vi "App - analyze RUS V6.vi"() -> ()   [LabVIEW 2018] (continued)
"file name str"="D:\\Data\\Ultrasound\\LSCO\\LSCO22__130814c\\5_Cooling_2nd_try\\September_2014\\091814\\14.56800K_500_2500_2.10000V_0.00000T_Sep18-2014__00-30-29_001_091814.bin", "mod time(min)"=58230990.483333334, "file format"=enum."binary", "power(V)"=2.1, "Magn Field(T) "=0.0}, {"temperature"=14.564, "temperature str"="14.56400", "file path"=path "D:/Data/Ultrasound/LSCO/LSCO22__130814c/5_Cooling_2nd_try/September_2014/091814/14.56400K_500_2500_2.10000V_0.00000T_Sep18-2014__00-31-48_001_091814.bin", "last mod"=timestamp(3493859508 s since 1904-01-01), "file name str"="D:\\Data\\Ultrasound\\LSCO\\LSCO22__130814c\\5_Cooling_2nd_try\\September_2014\\091814\\14.56400K_500_2500_2.10000V_0.00000T_Sep18-2014__00-31-48_001_091814.bin", "mod time(min)"=58230991.8, "file format"=enum."binary", "power(V)"=2.1, "Magn Field(T) "=0.0}, {"temperature"=14.565, "temperature str"="14.56500", "file path"=path "D:/Data/Ultrasound/LSCO/LSCO22__130814c/5_Cooling_2nd_try/September_2014/091814/14.56500K_500_2500_2.10000V_0.00000T_Sep18-2014__00-33-08_001_091814.bin", "last mod"=timestamp(3493859588 s since 1904-01-01), "file name str"="D:\\Data\\Ultrasound\\LSCO\\LSCO22__130814c\\5_Cooling_2nd_try\\September_2014\\091814\\14.56500K_500_2500_2.10000V_0.00000T_Sep18-2014__00-33-08_001_091814.bin", "mod time(min)"=58230993.13333333, "file format"=enum."binary", "power(V)"=2.1, "Magn Field(T) "=0.0}, {"temperature"=14.561, "temperature str"="14.56100", "file path"=path "D:/Data/Ultrasound/LSCO/LSCO22__130814c/5_Cooling_2nd_try/September_2014/091814/14.56100K_500_2500_2.10000V_0.00000T_Sep18-2014__00-34-27_001_091814.bin", "last mod"=timestamp(3493859667 s since 1904-01-01), "file name str"="D:\\Data\\Ultrasound\\LSCO\\LSCO22__130814c\\5_Cooling_2nd_try\\September_2014\\091814\\14.56100K_500_2500_2.10000V_0.00000T_Sep18-2014__00-34-27_001_091814.bin", "mod time(min)"=58230994.45, "file format"=enum."binary", "power(V)"=2.1, "Magn Field(T) "=0.0}, {"temperature"=14.557, "temperature str"="14.55700", "file path"=path "D:/Data/Ultrasound/LSCO/LSCO22__130814c/5_Cooling_2nd_try/September_2014/091814/14.55700K_500_2500_2.10000V_0.00000T_Sep18-2014__00-35-47_001_091814.bin", "last mod"=timestamp(3493859747 s since 1904-01-01), "file name str"="D:\\Data\\Ultrasound\\LSCO\\LSCO22__130814c\\5_Cooling_2nd_try\\September_2014\\091814\\14.55700K_500_2500_2.10000V_0.00000T_Sep18-2014__00-35-47_001_091814.bin", "mod time(min)"=58230995.78333333, "file format"=enum."binary", "power(V)"=2.1, "Magn Field(T) "=0.0}, {"temperature"=14.553, "temperature str"="14.55300", "file path"=path "D:/Data/Ultrasound/LSCO/LSCO22__130814c/5_Cooling_2nd_try/September_2014/091814/14.55300K_500_2500_2.10000V_0.00000T_Sep18-2014__00-37-06_001_091814.bin", "last mod"=timestamp(3493859826 s since 1904-01-01), "file name str"="D:\\Data\\Ultrasound\\LSCO\\LSCO22__130814c\\5_Cooling_2nd_try\\September_2014\\091814\\14.55300K_500_2500_2.10000V_0.00000T_Sep18-2014__00-37-06_001_091814.bin", "mod time(min)"=58230997.1, "file format"=enum."binary", "power(V)"=2.1, "Magn Field(T) "=0.0}, {"temperature"=14.55, "temperature str"="14.55000", "file path"=path "D:/Data/Ultrasound/LSCO/LSCO22__130814c/5_Cooling_2nd_try/September_2014/091814/14.55000K_500_2500_2.10000V_0.00000T_Sep18-2014__00-38-25_001_091814.bin", "last mod"=timestamp(3493859905 s since 1904-01-01), "file name str"="D:\\Data\\Ultrasound\\LSCO\\LSCO22__130814c\\5_Cooling_2nd_try\\September_2014\\091814\\14.55000K_500_2500_2.10000V_0.00000T_Sep18-2014__00-38-25_001_091814.bin", "mod time(min)"=58230998.416666664, "file format"=enum."binary", "power(V)"=2.1, "Magn Field(T) "=0.0}, {"temperature"=14.546, "temperature str"="14.54600", "file path"=path "D:/Data/Ultrasound/LSCO/LSCO22__130814c/5_Cooling_2nd_try/September_2014/091814/14.54600K_500_2500_2.10000V_0.00000T_Sep18-2014__00-39-45_001_091814.bin", "last mod"=timestamp(3493859985 s since 1904-01-01), "file name str"="D:\\Data\\Ultrasound\\LSCO\\LSCO22__130814c\\5_Cooling_2nd_try\\September_2014\\091814\\14.54600K_500_2500_2.10000V_0.00000T_Sep18-2014__00-39-45_001_091814.bin", "mod time(min)"=58230999.75, "file format"=enum."binary", "power(V)"=2.1, "Magn Field(T) "=0.0}, {"temperature"=14.543, "temperature str"="14.54300", "file path"=path "D:/Data/Ultrasound/LSCO/LSCO22__130814c/5_Cooling_2nd_try/September_2014/091814/14.54300K_500_2500_2.10000V_0.00000T_Sep18-2014__00-41-04_001_091814.bin", "last mod"=timestamp(3493860064 s since 1904-01-01), "file name str"="D:\\Data\\Ultrasound\\LSCO\\LSCO22__130814c\\5_Cooling_2nd_try\\September_2014\\091814\\14.54300K_500_2500_2.10000V_0.00000T_Sep18-2014__00-41-04_001_091814.bin", "mod time(min)"=58231001.06666667, "file format"=enum."binary", "power(V)"=2.1, "Magn Field(T) "=0.0}, {"temperature"=14.545, "temperature str"="14.54500", "file path"=path "D:/Data/Ultrasound/LSCO/LSCO22__130814c/5_Cooling_2nd_try/September_2014/091814/14.54500K_500_2500_2.10000V_0.00000T_Sep18-2014__00-42-24_001_091814.bin", "last mod"=timestamp(3493860144 s since 1904-01-01), "file name str"="D:\\Data\\Ultrasound\\LSCO\\LSCO22__130814c\\5_Cooling_2nd_try\\September_2014\\091814\\14.54500K_500_2500_2.10000V_0.00000T_Sep18-2014__00-42-24_001_091814.bin", "mod time(min)"=58231002.4, "file format"=enum."binary", "power(V)"=2.1, "Magn Field(T) "=0.0}, {"temperature"=14.546, "temperature str"="14.54600", "file path"=path "D:/Data/Ultrasound/LSCO/LSCO22__130814c/5_Cooling_2nd_try/September_2014/091814/14.54600K_500_2500_2.10000V_0.00000T_Sep18-2014__00-43-43_001_091814.bin", "last mod"=timestamp(3493860223 s since 1904-01-01), "file name str"="D:\\Data\\Ultrasound\\LSCO\\LSCO22__130814c\\5_Cooling_2nd_try\\September_2014\\091814\\14.54600K_500_2500_2.10000V_0.00000T_Sep18-2014__00-43-43_001_091814.bin", "mod time(min)"=58231003.71666667, "file format"=enum."binary", "power(V)"=2.1, "Magn Field(T) "=0.0}, {"temperature"=14.542, "temperature str"="14.54200", "file path"=path "D:/Data/Ultrasound/LSCO/LSCO22__130814c/5_Cooling_2nd_try/September_2014/091814/14.54200K_500_2500_2.10000V_0.00000T_Sep18-2014__00-45-02_001_091814.bin", "last mod"=timestamp(3493860302 s since 1904-01-01), "file name str"="D:\\Data\\Ultrasound\\LSCO\\LSCO22__130814c\\5_Cooling_2nd_try\\September_2014\\091814\\14.54200K_500_2500_2.10000V_0.00000T_Sep18-2014__00-45-02_001_091814.bin", "mod time(min)"=58231005.03333333, "file format"=enum."binary", "power(V)"=2.1, "Magn Field(T) "=0.0}, {"temperature"=14.545, "temperature str"="14.54500", "file path"=path "D:/Data/Ultrasound/LSCO/LSCO22__130814c/5_Cooling_2nd_try/September_2014/091814/14.54500K_500_2500_2.10000V_0.00000T_Sep18-2014__00-46-22_001_091814.bin", "last mod"=timestamp(3493860382 s since 1904-01-01), "file name str"="D:\\Data\\Ultrasound\\LSCO\\LSCO22__130814c\\5_Cooling_2nd_try\\September_2014\\091814\\14.54500K_500_2500_2.10000V_0.00000T_Sep18-2014__00-46-22_001_091814.bin", "mod time(min)"=58231006.36666667, "file format"=enum."binary", "power(V)"=2.1, "Magn Field(T) "=0.0}, {"temperature"=14.547, "temperature str"="14.54700", "file path"=path "D:/Data/Ultrasound/LSCO/LSCO22__130814c/5_Cooling_2nd_try/September_2014/091814/14.54700K_500_2500_2.10000V_0.00000T_Sep18-2014__00-47-41_001_091814.bin", "last mod"=timestamp(3493860461 s since 1904-01-01), "file name str"="D:\\Data\\Ultrasound\\LSCO\\LSCO22__130814c\\5_Cooling_2nd_try\\September_2014\\091814\\14.54700K_500_2500_2.10000V_0.00000T_Sep18-2014__00-47-41_001_091814.bin", "mod time(min)"=58231007.68333333, "file format"=enum."binary", "power(V)"=2.1, "Magn Field(T) "=0.0}, {"temperature"=14.544, "temperature str"="14.54400", "file path"=path "D:/Data/Ultrasound/LSCO/LSCO22__130814c/5_Cooling_2nd_try/September_2014/091814/14.54400K_500_2500_2.10000V_0.00000T_Sep18-2014__00-49-00_001_091814.bin", "last mod"=timestamp(3493860540 s since 1904-01-01), "file name str"="D:\\Data\\Ultrasound\\LSCO\\LSCO22__130814c\\5_Cooling_2nd_try\\September_2014\\091814\\14.54400K_500_2500_2.10000V_0.00000T_Sep18-2014__00-49-00_001_091814.bin", "mod time(min)"=58231009.0, "file format"=enum."binary", "power(V)"=2.1, "Magn Field(T) "=0.0}, {"temperature"=14.538, "temperature str"="14.53800", "file path"=path "D:/Data/Ultrasound/LSCO/LSCO22__130814c/5_Cooling_2nd_try/September_2014/091814/14.53800K_500_2500_2.10000V_0.00000T_Sep18-2014__00-50-20_001_091814.bin", "last mod"=timestamp(3493860620 s since 1904-01-01), "file name str"="D:\\Data\\Ultrasound\\LSCO\\LSCO22__130814c\\5_Cooling_2nd_try\\September_2014\\091814\\14.53800K_500_2500_2.10000V_0.00000T_Sep18-2014__00-50-20_001_091814.bin", "mod time(min)"=58231010.333333336, "file format"=enum."binary", "power(V)"=2.1, "Magn Field(T) "=0.0}, {"temperature"=14.537, "temperature str"="14.53700", "file path"=path "D:/Data/Ultrasound/LSCO/LSCO22__130814c/5_Cooling_2nd_try/September_2014/091814/14.53700K_500_2500_2.10000V_0.00000T_Sep18-2014__00-51-39_001_091814.bin", "last mod"=timestamp(3493860699 s since 1904-01-01), "file name str"="D:\\Data\\Ultrasound\\LSCO\\LSCO22__130814c\\5_Cooling_2nd_try\\September_2014\\091814\\14.53700K_500_2500_2.10000V_0.00000T_Sep18-2014__00-51-39_001_091814.bin", "mod time(min)"=58231011.65, "file format"=enum."binary", "power(V)"=2.1, "Magn Field(T) "=0.0}, {"temperature"=14.527, "temperature str"="14.52700", "file path"=path "D:/Data/Ultrasound/LSCO/LSCO22__130814c/5_Cooling_2nd_try/September_2014/091814/14.52700K_500_2500_2.10000V_0.00000T_Sep18-2014__00-52-59_001_091814.bin", "last mod"=timestamp(3493860779 s since 1904-01-01), "file name str"="D:\\Data\\Ultrasound\\LSCO\\LSCO22__130814c\\5_Cooling_2nd_try\\September_2014\\091814\\14.52700K_500_2500_2.10000V_0.00000T_Sep18-2014__00-52-59_001_091814.bin", "mod time(min)"=58231012.983333334, "file format"=enum."binary", "power(V)"=2.1, "Magn Field(T) "=0.0}, {"temperature"=14.532, "temperature str"="14.53200", "file path"=path "D:/Data/Ultrasound/LSCO/LSCO22__130814c/5_Cooling_2nd_try/September_2014/091814/14.53200K_500_2500_2.10000V_0.00000T_Sep18-2014__00-54-18_001_091814.bin", "last mod"=timestamp(3493860858 s since 1904-01-01), "file name str"="D:\\Data\\Ultrasound\\LSCO\\LSCO22__130814c\\5_Cooling_2nd_try\\September_2014\\091814\\14.53200K_500_2500_2.10000V_0.00000T_Sep18-2014__00-54-18_001_091814.bin", "mod time(min)"=58231014.3, "file format"=enum."binary", "power(V)"=2.1, "Magn Field(T) "=0.0}, {"temperature"=14.532, "temperature str"="14.53200", "file path"=path "D:/Data/Ultrasound/LSCO/LSCO22__130814c/5_Cooling_2nd_try/September_2014/091814/14.53200K_500_2500_2.10000V_0.00000T_Sep18-2014__00-55-37_001_091814.bin", "last mod"=timestamp(3493860937 s since 1904-01-01), "file name str"="D:\\Data\\Ultrasound\\LSCO\\LSCO22__130814c\\5_Cooling_2nd_try\\September_2014\\091814\\14.53200K_500_2500_2.10000V_0.00000T_Sep18-2014__00-55-37_001_091814.bin", "mod time(min)"=58231015.61666667, "file format"=enum."binary", "power(V)"=2.1, "Magn Field(T) "=0.0}, {"temperature"=14.525, "temperature str"="14.52500", "file path"=path "D:/Data/Ultrasound/LSCO/LSCO22__130814c/5_Cooling_2nd_try/September_2014/091814/14.52500K_500_2500_2.10000V_0.00000T_Sep18-2014__00-56-57_001_091814.bin", "last mod"=timestamp(3493861017 s since 1904-01-01), "file name str"="D:\\Data\\Ultrasound\\LSCO\\LSCO22__130814c\\5_Cooling_2nd_try\\September_2014\\091814\\14.52500K_500_2500_2.10000V_0.00000T_Sep18-2014__00-56-57_001_091814.bin", "mod time(min)"=58231016.95, "file format"=enum."binary", "power(V)"=2.1, "Magn Field(T) "=0.0}, {"temperature"=14.52, "temperature str"="14.52000", "file path"=path "D:/Data/Ultrasound/LSCO/LSCO22__130814c/5_Cooling_2nd_try/September_2014/091814/14.52000K_500_2500_2.10000V_0.00000T_Sep18-2014__00-58-16_001_091814.bin", "last mod"=timestamp(3493861096 s since 1904-01-01), "file name str"="D:\\Data\\Ultrasound\\LSCO\\LSCO22__130814c\\5_Cooling_2nd_try\\September_2014\\091814\\14.52000K_500_2500_2.10000V_0.00000T_Sep18-2014__00-58-16_001_091814.bin", "mod time(min)"=58231018.266666666, "file format"=enum."binary", "power(V)"=2.1, "Magn Field(T) "=0.0}, {"temperature"=14.519, "temperature str"="14.51900", "file path"=path "D:/Data/Ultrasound/LSCO/LSCO22__130814c/5_Cooling_2nd_try/September_2014/091814/14.51900K_500_2500_2.10000V_0.00000T_Sep18-2014__00-59-35_001_091814.bin", "last mod"=timestamp(3493861175 s since 1904-01-01), "file name str"="D:\\Data\\Ultrasound\\LSCO\\LSCO22__130814c\\5_Cooling_2nd_try\\September_2014\\091814\\14.51900K_500_2500_2.10000V_0.00000T_Sep18-2014__00-59-35_001_091814.bin", "mod time(min)"=58231019.583333336, "file format"=enum."binary", "power(V)"=2.1, "Magn Field(T) "=0.0}, {"temperature"=14.515, "temperature str"="14.51500", "file path"=path "D:/Data/Ultrasound/LSCO/LSCO22__130814c/5_Cooling_2nd_try/September_2014/091814/14.51500K_500_2500_2.10000V_0.00000T_Sep18-2014__01-00-55_001_091814.bin", "last mod"=timestamp(3493861255 s since 1904-01-01), "file name str"="D:\\Data\\Ultrasound\\LSCO\\LSCO22__130814c\\5_Cooling_2nd_try\\September_2014\\091814\\14.51500K_500_2500_2.10000V_0.00000T_Sep18-2014__01-00-55_001_091814.bin", "mod time(min)"=58231020.916666664, "file format"=enum."binary", "power(V)"=2.1, "Magn Field(T) "=0.0}, {"temperature"=14.515, "temperature str"="14.51500", "file path"=path "D:/Data/Ultrasound/LSCO/LSCO22__130814c/5_Cooling_2nd_try/September_2014/091814/14.51500K_500_2500_2.10000V_0.00000T_Sep18-2014__01-02-14_001_091814.bin", "last mod"=timestamp(3493861334 s since 1904-01-01), "file name str"="D:\\Data\\Ultrasound\\LSCO\\LSCO22__130814c\\5_Cooling_2nd_try\\September_2014\\091814\\14.51500K_500_2500_2.10000V_0.00000T_Sep18-2014__01-02-14_001_091814.bin", "mod time(min)"=58231022.233333334, "file format"=enum."binary", "power(V)"=2.1, "Magn Field(T) "=0.0}, {"temperature"=14.511, "temperature str"="14.51100", "file path"=path "D:/Data/Ultrasound/LSCO/LSCO22__130814c/5_Cooling_2nd_try/September_2014/091814/14.51100K_500_2500_2.10000V_0.00000T_Sep18-2014__01-03-34_001_091814.bin", "last mod"=timestamp(3493861414 s since 1904-01-01), "file name str"="D:\\Data\\Ultrasound\\LSCO\\LSCO22__130814c\\5_Cooling_2nd_try\\September_2014\\091814\\14.51100K_500_2500_2.10000V_0.00000T_Sep18-2014__01-03-34_001_091814.bin", "mod time(min)"=58231023.56666667, "file format"=enum."binary", "power(V)"=2.1, "Magn Field(T) "=0.0}, {"temperature"=14.506, "temperature str"="14.50600", "file path"=path "D:/Data/Ultrasound/LSCO/LSCO22__130814c/5_Cooling_2nd_try/September_2014/091814/14.50600K_500_2500_2.10000V_0.00000T_Sep18-2014__01-04-53_001_091814.bin", "last mod"=timestamp(3493861493 s since 1904-01-01), "file name str"="D:\\Data\\Ultrasound\\LSCO\\LSCO22__130814c\\5_Cooling_2nd_try\\September_2014\\091814\\14.50600K_500_2500_2.10000V_0.00000T_Sep18-2014__01-04-53_001_091814.bin", "mod time(min)"=58231024.88333333, "file format"=enum."binary", "power(V)"=2.1, "Magn Field(T) "=0.0}, {"temperature"=14.507, "temperature str"="14.50700", "file path"=path "D:/Data/Ultrasound/LSCO/LSCO22__130814c/5_Cooling_2nd_try/September_2014/091814/14.50700K_500_2500_2.10000V_0.00000T_Sep18-2014__01-06-12_001_091814.bin", "last mod"=timestamp(3493861572 s since 1904-01-01), "file name str"="D:\\Data\\Ultrasound\\LSCO\\LSCO22__130814c\\5_Cooling_2nd_try\\September_2014\\091814\\14.50700K_500_2500_2.10000V_0.00000T_Sep18-2014__01-06-12_001_091814.bin", "mod time(min)"=58231026.2, "file format"=enum."binary", "power(V)"=2.1, "Magn Field(T) "=0.0}, {"temperature"=14.503, "temperature str"="14.50300", "file path"=path "D:/Data/Ultrasound/LSCO/LSCO22__130814c/5_Cooling_2nd_try/September_2014/091814/14.50300K_500_2500_2.10000V_0.00000T_Sep18-2014__01-07-32_001_091814.bin", "last mod"=timestamp(3493861652 s since 1904-01-01), "file name str"="D:\\Data\\Ultrasound\\LSCO\\LSCO22__130814c\\5_Cooling_2nd_try\\September_2014\\091814\\14.50300K_500_2500_2.10000V_0.00000T_Sep18-2014__01-07-32_001_091814.bin", "mod time(min)"=58231027.53333333, "file format"=enum."binary", "power(V)"=2.1, "Magn Field(T) "=0.0}, {"temperature"=14.501, "temperature str"="14.50100", "file path"=path "D:/Data/Ultrasound/LSCO/LSCO22__130814c/5_Cooling_2nd_try/September_2014/091814/14.50100K_500_2500_2.10000V_0.00000T_Sep18-2014__01-08-51_001_091814.bin", "last mod"=timestamp(3493861731 s since 1904-01-01), "file name str"="D:\\Data\\Ultrasound\\LSCO\\LSCO22__130814c\\5_Cooling_2nd_try\\September_2014\\091814\\14.50100K_500_2500_2.10000V_0.00000T_Sep18-2014__01-08-51_001_091814.bin", "mod time(min)"=58231028.85, "file format"=enum."binary", "power(V)"=2.1, "Magn Field(T) "=0.0}, {"temperature"=14.5, "temperature str"="14.50000", "file path"=path "D:/Data/Ultrasound/LSCO/LSCO22__130814c/5_Cooling_2nd_try/September_2014/091814/14.50000K_500_2500_2.10000V_0.00000T_Sep18-2014__01-10-11_001_091814.bin", "last mod"=timestamp(3493861811 s since 1904-01-01), "file name str"="D:\\Data\\Ultrasound\\LSCO\\LSCO22__130814c\\5_Cooling_2nd_try\\September_2014\\091814\\14.50000K_500_2500_2.10000V_0.00000T_Sep18-2014__01-10-11_001_091814.bin", "mod time(min)"=58231030.18333333, "file format"=enum."binary", "power(V)"=2.1, "Magn Field(T) "=0.0}, {"temperature"=14.504, "temperature str"="14.50400", "file path"=path "D:/Data/Ultrasound/LSCO/LSCO22__130814c/5_Cooling_2nd_try/September_2014/091814/14.50400K_500_2500_2.10000V_0.00000T_Sep18-2014__01-11-30_001_091814.bin", "last mod"=timestamp(3493861890 s since 1904-01-01), "file name str"="D:\\Data\\Ultrasound\\LSCO\\LSCO22__130814c\\5_Cooling_2nd_try\\September_2014\\091814\\14.50400K_500_2500_2.10000V_0.00000T_Sep18-2014__01-11-30_001_091814.bin", "mod time(min)"=58231031.5, "file format"=enum."binary", "power(V)"=2.1, "Magn Field(T) "=0.0}, {"temperature"=14.504, "temperature str"="14.50400", "file path"=path "D:/Data/Ultrasound/LSCO/LSCO22__130814c/5_Cooling_2nd_try/September_2014/091814/14.50400K_500_2500_2.10000V_0.00000T_Sep18-2014__01-12-49_001_091814.bin", "last mod"=timestamp(3493861969 s since 1904-01-01), "file name str"="D:\\Data\\Ultrasound\\LSCO\\LSCO22__130814c\\5_Cooling_2nd_try\\September_2014\\091814\\14.50400K_500_2500_2.10000V_0.00000T_Sep18-2014__01-12-49_001_091814.bin", "mod time(min)"=58231032.81666667, "file format"=enum."binary", "power(V)"=2.1, "Magn Field(T) "=0.0}, {"temperature"=14.507, "temperature str"="14.50700", "file path"=path "D:/Data/Ultrasound/LSCO/LSCO22__130814c/5_Cooling_2nd_try/September_2014/091814/14.50700K_500_2500_2.10000V_0.00000T_Sep18-2014__01-14-09_001_091814.bin", "last mod"=timestamp(3493862049 s since 1904-01-01), "file name str"="D:\\Data\\Ultrasound\\LSCO\\LSCO22__130814c\\5_Cooling_2nd_try\\September_2014\\091814\\14.50700K_500_2500_2.10000V_0.00000T_Sep18-2014__01-14-09_001_091814.bin", "mod time(min)"=58231034.15, "file format"=enum."binary", "power(V)"=2.1, "Magn Field(T) "=0.0}, {"temperature"=14.502, "temperature str"="14.50200", "file path"=path "D:/Data/Ultrasound/LSCO/LSCO22__130814c/5_Cooling_2nd_try/September_2014/091814/14.50200K_500_2500_2.10000V_0.00000T_Sep18-2014__01-15-28_001_091814.bin", "last mod"=timestamp(3493862128 s since 1904-01-01), "file name str"="D:\\Data\\Ultrasound\\LSCO\\LSCO22__130814c\\5_Cooling_2nd_try\\September_2014\\091814\\14.50200K_500_2500_2.10000V_0.00000T_Sep18-2014__01-15-28_001_091814.bin", "mod time(min)"=58231035.46666667, "file format"=enum."binary", "power(V)"=2.1, "Magn Field(T) "=0.0}, {"temperature"=14.501, "temperature str"="14.50100", "file path"=path "D:/Data/Ultrasound/LSCO/LSCO22__130814c/5_Cooling_2nd_try/September_2014/091814/14.50100K_500_2500_2.10000V_0.00000T_Sep18-2014__01-16-47_001_091814.bin", "last mod"=timestamp(3493862207 s since 1904-01-01), "file name str"="D:\\Data\\Ultrasound\\LSCO\\LSCO22__130814c\\5_Cooling_2nd_try\\September_2014\\091814\\14.50100K_500_2500_2.10000V_0.00000T_Sep18-2014__01-16-47_001_091814.bin", "mod time(min)"=58231036.78333333, "file format"=enum."binary", "power(V)"=2.1, "Magn Field(T) "=0.0}, {"temperature"=14.503, "temperature str"="14.50300", "file path"=path "D:/Data/Ultrasound/LSCO/LSCO22__130814c/5_Cooling_2nd_try/September_2014/091814/14.50300K_500_2500_2.10000V_0.00000T_Sep18-2014__01-18-07_001_091814.bin", "last mod"=timestamp(3493862287 s since 1904-01-01), "file name str"="D:\\Data\\Ultrasound\\LSCO\\LSCO22__130814c\\5_Cooling_2nd_try\\September_2014\\091814\\14.50300K_500_2500_2.10000V_0.00000T_Sep18-2014__01-18-07_001_091814.bin", "mod time(min)"=58231038.11666667, "file format"=enum."binary", "power(V)"=2.1, "Magn Field(T) "=0.0}, {"temperature"=14.496, "temperature str"="14.49600", "file path"=path "D:/Data/Ultrasound/LSCO/LSCO22__130814c/5_Cooling_2nd_try/September_2014/091814/14.49600K_500_2500_2.10000V_0.00000T_Sep18-2014__01-19-26_001_091814.bin", "last mod"=timestamp(3493862366 s since 1904-01-01), "file name str"="D:\\Data\\Ultrasound\\LSCO\\LSCO22__130814c\\5_Cooling_2nd_try\\September_2014\\091814\\14.49600K_500_2500_2.10000V_0.00000T_Sep18-2014__01-19-26_001_091814.bin", "mod time(min)"=58231039.43333333, "file format"=enum."binary", "power(V)"=2.1, "Magn Field(T) "=0.0}, {"temperature"=14.494, "temperature str"="14.49400", "file path"=path "D:/Data/Ultrasound/LSCO/LSCO22__130814c/5_Cooling_2nd_try/September_2014/091814/14.49400K_500_2500_2.10000V_0.00000T_Sep18-2014__01-20-46_001_091814.bin", "last mod"=timestamp(3493862446 s since 1904-01-01), "file name str"="D:\\Data\\Ultrasound\\LSCO\\LSCO22__130814c\\5_Cooling_2nd_try\\September_2014\\091814\\14.49400K_500_2500_2.10000V_0.00000T_Sep18-2014__01-20-46_001_091814.bin", "mod time(min)"=58231040.766666666, "file format"=enum."binary", "power(V)"=2.1, "Magn Field(T) "=0.0}, {"temperature"=14.494, "temperature str"="14.49400", "file path"=path "D:/Data/Ultrasound/LSCO/LSCO22__130814c/5_Cooling_2nd_try/September_2014/091814/14.49400K_500_2500_2.10000V_0.00000T_Sep18-2014__01-22-05_001_091814.bin", "last mod"=timestamp(3493862525 s since 1904-01-01), "file name str"="D:\\Data\\Ultrasound\\LSCO\\LSCO22__130814c\\5_Cooling_2nd_try\\September_2014\\091814\\14.49400K_500_2500_2.10000V_0.00000T_Sep18-2014__01-22-05_001_091814.bin", "mod time(min)"=58231042.083333336, "file format"=enum."binary", "power(V)"=2.1, "Magn Field(T) "=0.0}, {"temperature"=14.485, "temperature str"="14.48500", "file path"=path "D:/Data/Ultrasound/LSCO/LSCO22__130814c/5_Cooling_2nd_try/September_2014/091814/14.48500K_500_2500_2.10000V_0.00000T_Sep18-2014__01-23-24_001_091814.bin", "last mod"=timestamp(3493862604 s since 1904-01-01), "file name str"="D:\\Data\\Ultrasound\\LSCO\\LSCO22__130814c\\5_Cooling_2nd_try\\September_2014\\091814\\14.48500K_500_2500_2.10000V_0.00000T_Sep18-2014__01-23-24_001_091814.bin", "mod time(min)"=58231043.4, "file format"=enum."binary", "power(V)"=2.1, "Magn Field(T) "=0.0}, {"temperature"=14.485, "temperature str"="14.48500", "file path"=path "D:/Data/Ultrasound/LSCO/LSCO22__130814c/5_Cooling_2nd_try/September_2014/091814/14.48500K_500_2500_2.10000V_0.00000T_Sep18-2014__01-24-44_001_091814.bin", "last mod"=timestamp(3493862684 s since 1904-01-01), "file name str"="D:\\Data\\Ultrasound\\LSCO\\LSCO22__130814c\\5_Cooling_2nd_try\\September_2014\\091814\\14.48500K_500_2500_2.10000V_0.00000T_Sep18-2014__01-24-44_001_091814.bin", "mod time(min)"=58231044.733333334, "file format"=enum."binary", "power(V)"=2.1, "Magn Field(T) "=0.0}, {"temperature"=14.487, "temperature str"="14.48700", "file path"=path "D:/Data/Ultrasound/LSCO/LSCO22__130814c/5_Cooling_2nd_try/September_2014/091814/14.48700K_500_2500_2.10000V_0.00000T_Sep18-2014__01-26-03_001_091814.bin", "last mod"=timestamp(3493862763 s since 1904-01-01), "file name str"="D:\\Data\\Ultrasound\\LSCO\\LSCO22__130814c\\5_Cooling_2nd_try\\September_2014\\091814\\14.48700K_500_2500_2.10000V_0.00000T_Sep18-2014__01-26-03_001_091814.bin", "mod time(min)"=58231046.05, "file format"=enum."binary", "power(V)"=2.1, "Magn Field(T) "=0.0}, {"temperature"=14.486, "temperature str"="14.48600", "file path"=path "D:/Data/Ultrasound/LSCO/LSCO22__130814c/5_Cooling_2nd_try/September_2014/091814/14.48600K_500_2500_2.10000V_0.00000T_Sep18-2014__01-27-22_001_091814.bin", "last mod"=timestamp(3493862842 s since 1904-01-01), "file name str"="D:\\Data\\Ultrasound\\LSCO\\LSCO22__130814c\\5_Cooling_2nd_try\\September_2014\\091814\\14.48600K_500_2500_2.10000V_0.00000T_Sep18-2014__01-27-22_001_091814.bin", "mod time(min)"=58231047.36666667, "file format"=enum."binary", "power(V)"=2.1, "Magn Field(T) "=0.0}, {"temperature"=14.479, "temperature str"="14.47900", "file path"=path "D:/Data/Ultrasound/LSCO/LSCO22__130814c/5_Cooling_2nd_try/September_2014/091814/14.47900K_500_2500_2.10000V_0.00000T_Sep18-2014__01-28-42_001_091814.bin", "last mod"=timestamp(3493862922 s since 1904-01-01), "file name str"="D:\\Data\\Ultrasound\\LSCO\\LSCO22__130814c\\5_Cooling_2nd_try\\September_2014\\091814\\14.47900K_500_2500_2.10000V_0.00000T_Sep18-2014__01-28-42_001_091814.bin", "mod time(min)"=58231048.7, "file format"=enum."binary", "power(V)"=2.1, "Magn Field(T) "=0.0}, {"temperature"=14.477, "temperature str"="14.47700", "file path"=path "D:/Data/Ultrasound/LSCO/LSCO22__130814c/5_Cooling_2nd_try/September_2014/091814/14.47700K_500_2500_2.10000V_0.00000T_Sep18-2014__01-30-01_001_091814.bin", "last mod"=timestamp(3493863001 s since 1904-01-01), "file name str"="D:\\Data\\Ultrasound\\LSCO\\LSCO22__130814c\\5_Cooling_2nd_try\\September_2014\\091814\\14.47700K_500_2500_2.10000V_0.00000T_Sep18-2014__01-30-01_001_091814.bin", "mod time(min)"=58231050.016666666, "file format"=enum."binary", "power(V)"=2.1, "Magn Field(T) "=0.0}, {"temperature"=14.476, "temperature str"="14.47600", "file path"=path "D:/Data/Ultrasound/LSCO/LSCO22__130814c/5_Cooling_2nd_try/September_2014/091814/14.47600K_500_2500_2.10000V_0.00000T_Sep18-2014__01-31-21_001_091814.bin", "last mod"=timestamp(3493863081 s since 1904-01-01), "file name str"="D:\\Data\\Ultrasound\\LSCO\\LSCO22__130814c\\5_Cooling_2nd_try\\September_2014\\091814\\14.47600K_500_2500_2.10000V_0.00000T_Sep18-2014__01-31-21_001_091814.bin", "mod time(min)"=58231051.35, "file format"=enum."binary", "power(V)"=2.1, "Magn Field(T) "=0.0}, {"temperature"=14.474, "temperature str"="14.47400", "file path"=path "D:/Data/Ultrasound/LSCO/LSCO22__130814c/5_Cooling_2nd_try/September_2014/091814/14.47400K_500_2500_2.10000V_0.00000T_Sep18-2014__01-32-40_001_091814.bin", "last mod"=timestamp(3493863160 s since 1904-01-01), "file name str"="D:\\Data\\Ultrasound\\LSCO\\LSCO22__130814c\\5_Cooling_2nd_try\\September_2014\\091814\\14.47400K_500_2500_2.10000V_0.00000T_Sep18-2014__01-32-40_001_091814.bin", "mod time(min)"=58231052.666666664, "file format"=enum."binary", "power(V)"=2.1, "Magn Field(T) "=0.0}, {"temperature"=14.473, "temperature str"="14.47300", "file path"=path "D:/Data/Ultrasound/LSCO/LSCO22__130814c/5_Cooling_2nd_try/September_2014/091814/14.47300K_500_2500_2.10000V_0.00000T_Sep18-2014__01-33-59_001_091814.bin", "last mod"=timestamp(3493863239 s since 1904-01-01), "file name str"="D:\\Data\\Ultrasound\\LSCO\\LSCO22__130814c\\5_Cooling_2nd_try\\September_2014\\091814\\14.47300K_500_2500_2.10000V_0.00000T_Sep18-2014__01-33-59_001_091814.bin", "mod time(min)"=58231053.983333334, "file format"=enum."binary", "power(V)"=2.1, "Magn Field(T) "=0.0}, {"temperature"=14.478, "temperature str"="14.47800", "file path"=path "D:/Data/Ultrasound/LSCO/LSCO22__130814c/5_Cooling_2nd_try/September_2014/091814/14.47800K_500_2500_2.10000V_0.00000T_Sep18-2014__01-35-19_001_091814.bin", "last mod"=timestamp(3493863319 s since 1904-01-01), "file name str"="D:\\Data\\Ultrasound\\LSCO\\LSCO22__130814c\\5_Cooling_2nd_try\\September_2014\\091814\\14.47800K_500_2500_2.10000V_0.00000T_Sep18-2014__01-35-19_001_091814.bin", "mod time(min)"=58231055.31666667, "file format"=enum."binary", "power(V)"=2.1, "Magn Field(T) "=0.0}, {"temperature"=14.475, "temperature str"="14.47500", "file path"=path "D:/Data/Ultrasound/LSCO/LSCO22__130814c/5_Cooling_2nd_try/September_2014/091814/14.47500K_500_2500_2.10000V_0.00000T_Sep18-2014__01-36-38_001_091814.bin", "last mod"=timestamp(3493863398 s since 1904-01-01), "file name str"="D:\\Data\\Ultrasound\\LSCO\\LSCO22__130814c\\5_Cooling_2nd_try\\September_2014\\091814\\14.47500K_500_2500_2.10000V_0.00000T_Sep18-2014__01-36-38_001_091814.bin", "mod time(min)"=58231056.63333333, "file format"=enum."binary", "power(V)"=2.1, "Magn Field(T) "=0.0}, {"temperature"=14.47, "temperature str"="14.47000", "file path"=path "D:/Data/Ultrasound/LSCO/LSCO22__130814c/5_Cooling_2nd_try/September_2014/091814/14.47000K_500_2500_2.10000V_0.00000T_Sep18-2014__01-37-58_001_091814.bin", "last mod"=timestamp(3493863478 s since 1904-01-01), "file name str"="D:\\Data\\Ultrasound\\LSCO\\LSCO22__130814c\\5_Cooling_2nd_try\\September_2014\\091814\\14.47000K_500_2500_2.10000V_0.00000T_Sep18-2014__01-37-58_001_091814.bin", "mod time(min)"=58231057.96666667, "file format"=enum."binary", "power(V)"=2.1, "Magn Field(T) "=0.0}, {"temperature"=14.472, "temperature str"="14.47200", "file path"=path "D:/Data/Ultrasound/LSCO/LSCO22__130814c/5_Cooling_2nd_try/September_2014/091814/14.47200K_500_2500_2.10000V_0.00000T_Sep18-2014__01-39-17_001_091814.bin", "last mod"=timestamp(3493863557 s since 1904-01-01), "file name str"="D:\\Data\\Ultrasound\\LSCO\\LSCO22__130814c\\5_Cooling_2nd_try\\September_2014\\091814\\14.47200K_500_2500_2.10000V_0.00000T_Sep18-2014__01-39-17_001_091814.bin", "mod time(min)"=58231059.28333333, "file format"=enum."binary", "power(V)"=2.1, "Magn Field(T) "=0.0}, {"temperature"=14.471, "temperature str"="14.47100", "file path"=path "D:/Data/Ultrasound/LSCO/LSCO22__130814c/5_Cooling_2nd_try/September_2014/091814/14.47100K_500_2500_2.10000V_0.00000T_Sep18-2014__01-40-36_001_091814.bin", "last mod"=timestamp(3493863636 s since 1904-01-01), "file name str"="D:\\Data\\Ultrasound\\LSCO\\LSCO22__130814c\\5_Cooling_2nd_try\\September_2014\\091814\\14.47100K_500_2500_2.10000V_0.00000T_Sep18-2014__01-40-36_001_091814.bin", "mod time(min)"=58231060.6, "file format"=enum."binary", "power(V)"=2.1, "Magn Field(T) "=0.0}, {"temperature"=14.469, "temperature str"="14.46900", "file path"=path "D:/Data/Ultrasound/LSCO/LSCO22__130814c/5_Cooling_2nd_try/September_2014/091814/14.46900K_500_2500_2.10000V_0.00000T_Sep18-2014__01-41-56_001_091814.bin", "last mod"=timestamp(3493863716 s since 1904-01-01), "file name str"="D:\\Data\\Ultrasound\\LSCO\\LSCO22__130814c\\5_Cooling_2nd_try\\September_2014\\091814\\14.46900K_500_2500_2.10000V_0.00000T_Sep18-2014__01-41-56_001_091814.bin", "mod time(min)"=58231061.93333333, "file format"=enum."binary", "power(V)"=2.1, "Magn Field(T) "=0.0}, {"temperature"=14.466, "temperature str"="14.46600", "file path"=path "D:/Data/Ultrasound/LSCO/LSCO22__130814c/5_Cooling_2nd_try/September_2014/091814/14.46600K_500_2500_2.10000V_0.00000T_Sep18-2014__01-43-15_001_091814.bin", "last mod"=timestamp(3493863795 s since 1904-01-01), "file name str"="D:\\Data\\Ultrasound\\LSCO\\LSCO22__130814c\\5_Cooling_2nd_try\\September_2014\\091814\\14.46600K_500_2500_2.10000V_0.00000T_Sep18-2014__01-43-15_001_091814.bin", "mod time(min)"=58231063.25, "file format"=enum."binary", "power(V)"=2.1, "Magn Field(T) "=0.0}, {"temperature"=14.467, "temperature str"="14.46700", "file path"=path "D:/Data/Ultrasound/LSCO/LSCO22__130814c/5_Cooling_2nd_try/September_2014/091814/14.46700K_500_2500_2.10000V_0.00000T_Sep18-2014__01-44-34_001_091814.bin", "last mod"=timestamp(3493863874 s since 1904-01-01), "file name str"="D:\\Data\\Ultrasound\\LSCO\\LSCO22__130814c\\5_Cooling_2nd_try\\September_2014\\091814\\14.46700K_500_2500_2.10000V_0.00000T_Sep18-2014__01-44-34_001_091814.bin", "mod time(min)"=58231064.56666667, "file format"=enum."binary", "power(V)"=2.1, "Magn Field(T) "=0.0}, {"temperature"=14.468, "temperature str"="14.46800", "file path"=path "D:/Data/Ultrasound/LSCO/LSCO22__130814c/5_Cooling_2nd_try/September_2014/091814/14.46800K_500_2500_2.10000V_0.00000T_Sep18-2014__01-45-54_001_091814.bin", "last mod"=timestamp(3493863954 s since 1904-01-01), "file name str"="D:\\Data\\Ultrasound\\LSCO\\LSCO22__130814c\\5_Cooling_2nd_try\\September_2014\\091814\\14.46800K_500_2500_2.10000V_0.00000T_Sep18-2014__01-45-54_001_091814.bin", "mod time(min)"=58231065.9, "file format"=enum."binary", "power(V)"=2.1, "Magn Field(T) "=0.0}, {"temperature"=14.463, "temperature str"="14.46300", "file path"=path "D:/Data/Ultrasound/LSCO/LSCO22__130814c/5_Cooling_2nd_try/September_2014/091814/14.46300K_500_2500_2.10000V_0.00000T_Sep18-2014__01-47-13_001_091814.bin", "last mod"=timestamp(3493864033 s since 1904-01-01), "file name str"="D:\\Data\\Ultrasound\\LSCO\\LSCO22__130814c\\5_Cooling_2nd_try\\September_2014\\091814\\14.46300K_500_2500_2.10000V_0.00000T_Sep18-2014__01-47-13_001_091814.bin", "mod time(min)"=58231067.21666667, "file format"=enum."binary", "power(V)"=2.1, "Magn Field(T) "=0.0}, {"temperature"=14.464, "temperature str"="14.46400", "file path"=path "D:/Data/Ultrasound/LSCO/LSCO22__130814c/5_Cooling_2nd_try/September_2014/091814/14.46400K_500_2500_2.10000V_0.00000T_Sep18-2014__01-48-33_001_091814.bin", "last mod"=timestamp(3493864113 s since 1904-01-01), "file name str"="D:\\Data\\Ultrasound\\LSCO\\LSCO22__130814c\\5_Cooling_2nd_try\\September_2014\\091814\\14.46400K_500_2500_2.10000V_0.00000T_Sep18-2014__01-48-33_001_091814.bin", "mod time(min)"=58231068.55, "file format"=enum."binary", "power(V)"=2.1, "Magn Field(T) "=0.0}, {"temperature"=14.462, "temperature str"="14.46200", "file path"=path "D:/Data/Ultrasound/LSCO/LSCO22__130814c/5_Cooling_2nd_try/September_2014/091814/14.46200K_500_2500_2.10000V_0.00000T_Sep18-2014__01-49-52_001_091814.bin", "last mod"=timestamp(3493864192 s since 1904-01-01), "file name str"="D:\\Data\\Ultrasound\\LSCO\\LSCO22__130814c\\5_Cooling_2nd_try\\September_2014\\091814\\14.46200K_500_2500_2.10000V_0.00000T_Sep18-2014__01-49-52_001_091814.bin", "mod time(min)"=58231069.86666667, "file format"=enum."binary", "power(V)"=2.1, "Magn Field(T) "=0.0}, {"temperature"=14.457, "temperature str"="14.45700", "file path"=path "D:/Data/Ultrasound/LSCO/LSCO22__130814c/5_Cooling_2nd_try/September_2014/091814/14.45700K_500_2500_2.10000V_0.00000T_Sep18-2014__01-51-11_001_091814.bin", "last mod"=timestamp(3493864271 s since 1904-01-01), "file name str"="D:\\Data\\Ultrasound\\LSCO\\LSCO22__130814c\\5_Cooling_2nd_try\\September_2014\\091814\\14.45700K_500_2500_2.10000V_0.00000T_Sep18-2014__01-51-11_001_091814.bin", "mod time(min)"=58231071.18333333, "file format"=enum."binary", "power(V)"=2.1, "Magn Field(T) "=0.0}, {"temperature"=14.457, "temperature str"="14.45700", "file path"=path "D:/Data/Ultrasound/LSCO/LSCO22__130814c/5_Cooling_2nd_try/September_2014/091814/14.45700K_500_2500_2.10000V_0.00000T_Sep18-2014__01-52-31_001_091814.bin", "last mod"=timestamp(3493864351 s since 1904-01-01), "file name str"="D:\\Data\\Ultrasound\\LSCO\\LSCO22__130814c\\5_Cooling_2nd_try\\September_2014\\091814\\14.45700K_500_2500_2.10000V_0.00000T_Sep18-2014__01-52-31_001_091814.bin", "mod time(min)"=58231072.516666666, "file format"=enum."binary", "power(V)"=2.1, "Magn Field(T) "=0.0}, {"temperature"=14.456, "temperature str"="14.45600", "file path"=path "D:/Data/Ultrasound/LSCO/LSCO22__130814c/5_Cooling_2nd_try/September_2014/091814/14.45600K_500_2500_2.10000V_0.00000T_Sep18-2014__01-53-50_001_091814.bin", "last mod"=timestamp(3493864430 s since 1904-01-01), "file name str"="D:\\Data\\Ultrasound\\LSCO\\LSCO22__130814c\\5_Cooling_2nd_try\\September_2014\\091814\\14.45600K_500_2500_2.10000V_0.00000T_Sep18-2014__01-53-50_001_091814.bin", "mod time(min)"=58231073.833333336, "file format"=enum."binary", "power(V)"=2.1, "Magn Field(T) "=0.0}, {"temperature"=14.45, "temperature str"="14.45000", "file path"=path "D:/Data/Ultrasound/LSCO/LSCO22__130814c/5_Cooling_2nd_try/September_2014/091814/14.45000K_500_2500_2.10000V_0.00000T_Sep18-2014__01-55-10_001_091814.bin", "last mod"=timestamp(3493864510 s since 1904-01-01), "file name str"="D:\\Data\\Ultrasound\\LSCO\\LSCO22__130814c\\5_Cooling_2nd_try\\September_2014\\091814\\14.45000K_500_2500_2.10000V_0.00000T_Sep18-2014__01-55-10_001_091814.bin", "mod time(min)"=58231075.166666664, "file format"=enum."binary", "power(V)"=2.1, "Magn Field(T) "=0.0}, {"temperature"=14.449, "temperature str"="14.44900", "file path"=path "D:/Data/Ultrasound/LSCO/LSCO22__130814c/5_Cooling_2nd_try/September_2014/091814/14.44900K_500_2500_2.10000V_0.00000T_Sep18-2014__01-56-29_001_091814.bin", "last mod"=timestamp(3493864589 s since 1904-01-01), "file name str"="D:\\Data\\Ultrasound\\LSCO\\LSCO22__130814c\\5_Cooling_2nd_try\\September_2014\\091814\\14.44900K_500_2500_2.10000V_0.00000T_Sep18-2014__01-56-29_001_091814.bin", "mod time(min)"=58231076.483333334, "file format"=enum."binary", "power(V)"=2.1, "Magn Field(T) "=0.0}, {"temperature"=14.446, "temperature str"="14.44600", "file path"=path "D:/Data/Ultrasound/LSCO/LSCO22__130814c/5_Cooling_2nd_try/September_2014/091814/14.44600K_500_2500_2.10000V_0.00000T_Sep18-2014__01-57-48_001_091814.bin", "last mod"=timestamp(3493864668 s since 1904-01-01), "file name str"="D:\\Data\\Ultrasound\\LSCO\\LSCO22__130814c\\5_Cooling_2nd_try\\September_2014\\091814\\14.44600K_500_2500_2.10000V_0.00000T_Sep18-2014__01-57-48_001_091814.bin", "mod time(min)"=58231077.8, "file format"=enum."binary", "power(V)"=2.1, "Magn Field(T) "=0.0}, {"temperature"=14.451, "temperature str"="14.45100", "file path"=path "D:/Data/Ultrasound/LSCO/LSCO22__130814c/5_Cooling_2nd_try/September_2014/091814/14.45100K_500_2500_2.10000V_0.00000T_Sep18-2014__01-59-08_001_091814.bin", "last mod"=timestamp(3493864748 s since 1904-01-01), "file name str"="D:\\Data\\Ultrasound\\LSCO\\LSCO22__130814c\\5_Cooling_2nd_try\\September_2014\\091814\\14.45100K_500_2500_2.10000V_0.00000T_Sep18-2014__01-59-08_001_091814.bin", "mod time(min)"=58231079.13333333, "file format"=enum."binary", "power(V)"=2.1, "Magn Field(T) "=0.0}, {"temperature"=14.451, "temperature str"="14.45100", "file path"=path "D:/Data/Ultrasound/LSCO/LSCO22__130814c/5_Cooling_2nd_try/September_2014/091814/14.45100K_500_2500_2.10000V_0.00000T_Sep18-2014__02-00-27_001_091814.bin", "last mod"=timestamp(3493864827 s since 1904-01-01), "file name str"="D:\\Data\\Ultrasound\\LSCO\\LSCO22__130814c\\5_Cooling_2nd_try\\September_2014\\091814\\14.45100K_500_2500_2.10000V_0.00000T_Sep18-2014__02-00-27_001_091814.bin", "mod time(min)"=58231080.45, "file format"=enum."binary", "power(V)"=2.1, "Magn Field(T) "=0.0}, {"temperature"=14.448, "temperature str"="14.44800", "file path"=path "D:/Data/Ultrasound/LSCO/LSCO22__130814c/5_Cooling_2nd_try/September_2014/091814/14.44800K_500_2500_2.10000V_0.00000T_Sep18-2014__02-01-46_001_091814.bin", "last mod"=timestamp(3493864906 s since 1904-01-01), "file name str"="D:\\Data\\Ultrasound\\LSCO\\LSCO22__130814c\\5_Cooling_2nd_try\\September_2014\\091814\\14.44800K_500_2500_2.10000V_0.00000T_Sep18-2014__02-01-46_001_091814.bin", "mod time(min)"=58231081.766666666, "file format"=enum."binary", "power(V)"=2.1, "Magn Field(T) "=0.0}, {"temperature"=14.449, "temperature str"="14.44900", "file path"=path "D:/Data/Ultrasound/LSCO/LSCO22__130814c/5_Cooling_2nd_try/September_2014/091814/14.44900K_500_2500_2.10000V_0.00000T_Sep18-2014__02-03-06_001_091814.bin", "last mod"=timestamp(3493864986 s since 1904-01-01), "file name str"="D:\\Data\\Ultrasound\\LSCO\\LSCO22__130814c\\5_Cooling_2nd_try\\September_2014\\091814\\14.44900K_500_2500_2.10000V_0.00000T_Sep18-2014__02-03-06_001_091814.bin", "mod time(min)"=58231083.1, "file format"=enum."binary", "power(V)"=2.1, "Magn Field(T) "=0.0}, {"temperature"=14.451, "temperature str"="14.45100", "file path"=path "D:/Data/Ultrasound/LSCO/LSCO22__130814c/5_Cooling_2nd_try/September_2014/091814/14.45100K_500_2500_2.10000V_0.00000T_Sep18-2014__02-04-25_001_091814.bin", "last mod"=timestamp(3493865065 s since 1904-01-01), "file name str"="D:\\Data\\Ultrasound\\LSCO\\LSCO22__130814c\\5_Cooling_2nd_try\\September_2014\\091814\\14.45100K_500_2500_2.10000V_0.00000T_Sep18-2014__02-04-25_001_091814.bin", "mod time(min)"=58231084.416666664, "file format"=enum."binary", "power(V)"=2.1, "Magn Field(T) "=0.0}, {"temperature"=14.449,
